vi "Get Table Configuration.vi"(8 "error in (no error)":errorcluster, 11 "Form from Table Configuration in":refnum<class "Form from Table Configuration.lvclass">) -> (0 "error out":errorcluster, 2 "Table Configuration":refnum<class "Table Configuration Interface.lvclass">, 3 "Form from Table Configuration out":refnum<class "Form from Table Configuration.lvclass">)   [LabVIEW 2020, in "Panel Form Controller.lvlib" / "Form from Table Configuration.lvclass"]
uses:
  Form from Table Configuration.lvclass
  Database OOP/Table Libraries/Table Configuration Interface/Table Configuration Interface.lvclass
  Controller Configuration/Panel Form Controller Configuration.lvclass
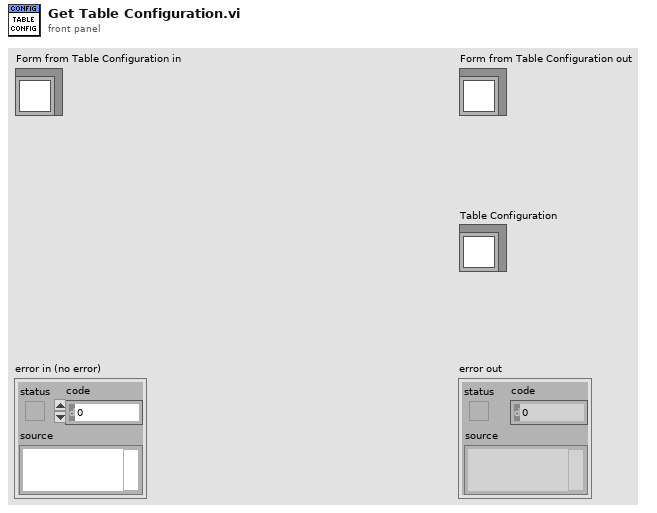
[diagram p1: front panel]
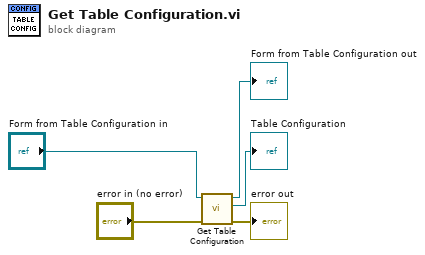
[diagram p0: block diagram]
diagram:
  n1 = call-parent "Get Table Configuration.vi"("error in (no error)"="error in (no error)", "Panel Form Controller Configuration in"="Form from Table Configuration in") -> ("error out"=→"error out":errorcluster, "Table Configuration"=→"Table Configuration":refnum<class "Table Configuration Interface.lvclass">, "Panel Form Controller Configuration out"=→"Form from Table Configuration out":refnum<class "Form from Table Configuration.lvclass">)  [unwired: 7 in]
